vi "Stop Core.vi"(10 "final error code":i32, 11 "National Instrument USB-6501 in":refnum<class "National Instrument USB-6501.lvclass">) -> (3 "National Instrument USB-6501 out":refnum<class "National Instrument USB-6501.lvclass">)   [LabVIEW 2014]
doc: "(<B>Filename</B>: Actor Framework.lvlib:Actor.lvclass:Stop Core.vi)\n\nDefines what the actor does before it stops. Use the <B>final error code</B> input to determine whether the actor shut down in response to an error.\n\nBy default, this method does nothing. A descendant class may override it to define behavior, such as shutting down any processes the actor initiated in its override of the Actor Core method."
uses:
  National Instrument USB-6501.lvclass
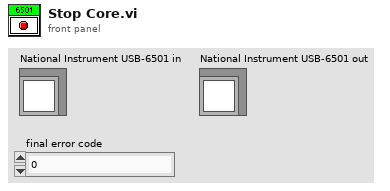
[diagram p1: front panel]
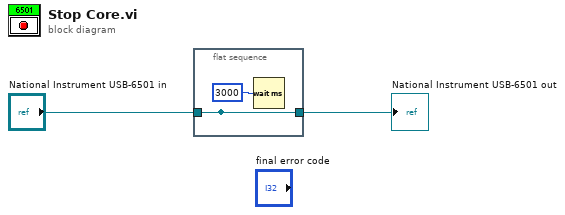
[diagram p0: block diagram]
diagram:
  n1 = flat-sequence {
    tunnel: [w3] -> _
    tunnel: "National Instrument USB-6501 in" -> [w3]
    tunnel: [w3] -> w1
    frame #0 {
      n2 = Wait (ms)(milliseconds to wait=u32 3000) -> ()  [unwired: 1 out]
    }
  }
  "National Instrument USB-6501 out" <- w1
